vi "Multiple Core CPUs.vi"   [LabVIEW 2014]
uses:
  <vilib>/Platform/TimedLoop/XDataNode/timing_clust.ctl
  <vilib>/Platform/TimedLoop/XDataNode/nitl_modes.ctl
  <vilib>/Platform/TimedLoop/XDataNode/wakeup.ctl
  <vilib>/platform/TimedLoop/XDataNode/XDataNode.xnode
  <vilib>/Platform/TimedLoop/XDataNode/XDNodeRunTimeDep.lvlib
types:
  T1 = typedef "XDNodeRunTimeDep.lvlib/timing_clust.ctl" = cluster{"Expected End [f-1]":u64, "Actual End [f-1]":u64, "Finished Late? [f-1]":bool, "Expected End [i-1]":u64, "Actual End [i-1]":u64, "Finished Late? [i-1]":bool, "Expected Start [i]":u64, "Actual Start [i]":u64, "Expected Start [f]":u64, "Actual Start [f]":u64, "Source Name":string, "Structure Name":string, "Period":i64, "Deadline":i64, "Offset":i64, "Start":i64, "Priority":i32, "Timeout":i32, "Mode":T2, "Wakeup Reason":T3, "Error":errorcluster, "Source Type":string, "Secondary Source Type":string, "Global End Time":u64, "Global Start Time":u64, "Frame Duration":u64, "Iteration Duration":u64, "Assigned CPU":i32, "I/O Scan Engine Mode":u32}
  T2 = typedef "XDNodeRunTimeDep.lvlib/nitl_modes.ctl" = enum32{"No Change", "Process missed periods, maintain original phase", "Discard missed periods, maintain original phase", "Process missed periods, ignore original phase", "Discard missed periods, ignore original phase"}
  T3 = typedef "XDNodeRunTimeDep.lvlib/wakeup.ctl" = enum32{"Normal", "Aborted", "Asynchronous wakeup", "Timing source error", "Timed loop error", "Timeout"}
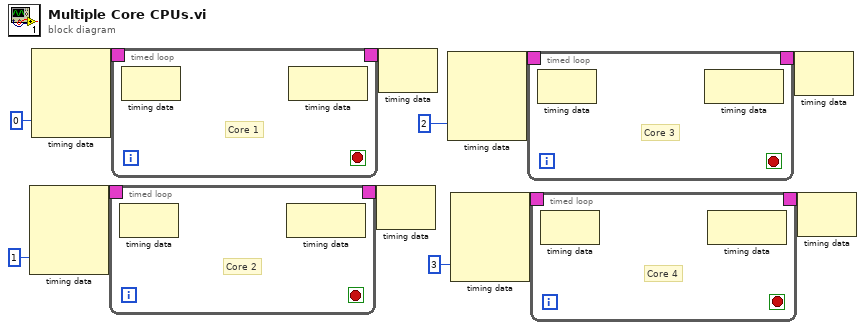
[diagram p0: block diagram]
diagram:
  n1 = node-c288(1 ("Processor")) -> (w9:T1)  [unwired: 3 in]
  n2 = node-c288(0 ("Processor")) -> (w12:T1)  [unwired: 3 in]
  n3 = timed-loop {
    timing: w9 -> [_]
    timing-out: [_] -> w8
    stop <- _ stop-if-true
    # "Core 2"
    n4 = node-c288() -> ()  [unwired: 1 in, 1 out]
    n5 = node-c288() -> ()  [unwired: 1 in, 1 out]
  }
  n6 = timed-loop {
    timing: w12 -> [_]
    timing-out: [_] -> w11
    stop <- _ stop-if-true
    # "Core 1"
    n7 = node-c288() -> ()  [unwired: 1 in, 1 out]
    n8 = node-c288() -> ()  [unwired: 1 in, 1 out]
  }
  n9 = node-c288(w8) -> ()  [unwired: 1 out]
  n10 = node-c288(w11) -> ()  [unwired: 1 out]
  n11 = node-c288(2 ("Processor")) -> (w7:T1)  [unwired: 3 in]
  n12 = node-c288(3 ("Processor")) -> (w5:T1)  [unwired: 3 in]
  n13 = timed-loop {
    timing: w7 -> [_]
    timing-out: [_] -> w6
    stop <- _ stop-if-true
    # "Core 3"
    n14 = node-c288() -> ()  [unwired: 1 in, 1 out]
    n15 = node-c288() -> ()  [unwired: 1 in, 1 out]
  }
  n16 = timed-loop {
    timing: w5 -> [_]
    timing-out: [_] -> w4
    stop <- _ stop-if-true
    # "Core 4"
    n17 = node-c288() -> ()  [unwired: 1 in, 1 out]
    n18 = node-c288() -> ()  [unwired: 1 in, 1 out]
  }
  n19 = node-c288(w6) -> ()  [unwired: 1 out]
  n20 = node-c288(w4) -> ()  [unwired: 1 out]
